vi "Sync.vi"(8 "Input Stream":dbl[](array[numeric]), 9 "error in (no error)":errorcluster, 10 "Frame Instruction":T1, 11 "PN sequence order (9)":i32=9) -> (0 "number 2":u32, 1 "number":u32, 2 "error out":errorcluster)   [LabVIEW 2014]
uses:
  <vilib>/addons/Modulation/Digital/General/MT Generate Bits (Galois, PN Order).vi
  <vilib>/addons/Modulation/Digital/Support/Common/Validators/mod_Generate Bits Validate.vi
  <vilib>/addons/Modulation/Analog/support/mod_Set Error Source.vi
  <vilib>/addons/Modulation/Digital/General/subVIs/mod_Generate Bits PN Sequence.vi
  <vilib>/addons/Modulation/niDMT.lvlib
panel:
  out "Numeric":dbl
  out "output bit stream":i8[](array[numeric])
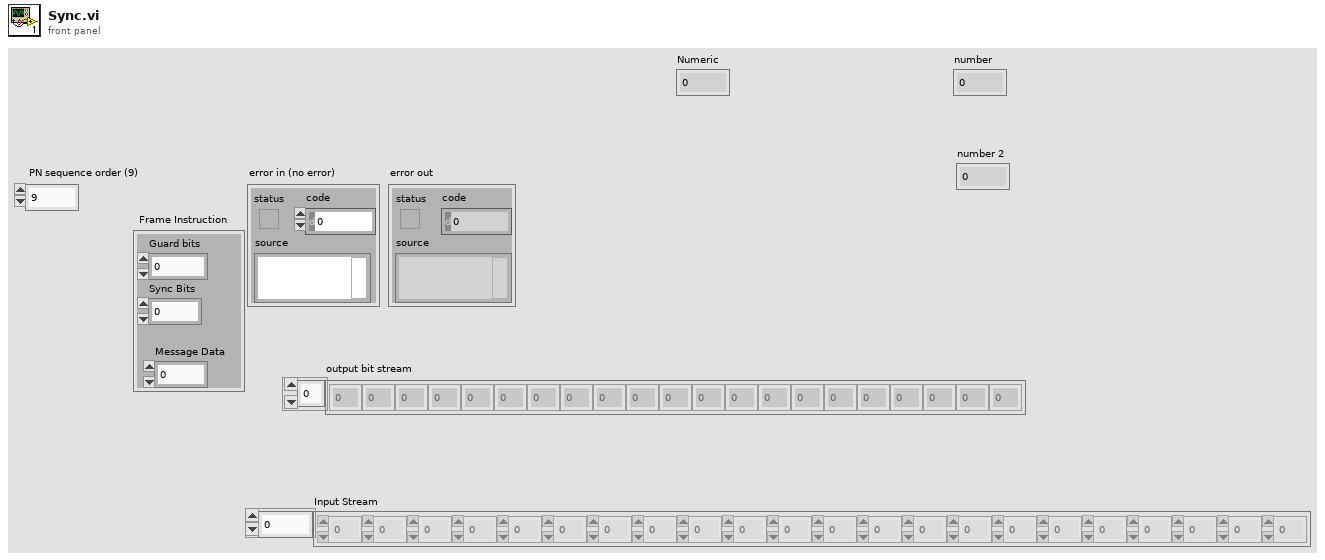
[diagram p1: front panel]
types:
  T1 = cluster{"Guard bits":dbl, "Sync Bits":dbl, "Message Data":dbl}
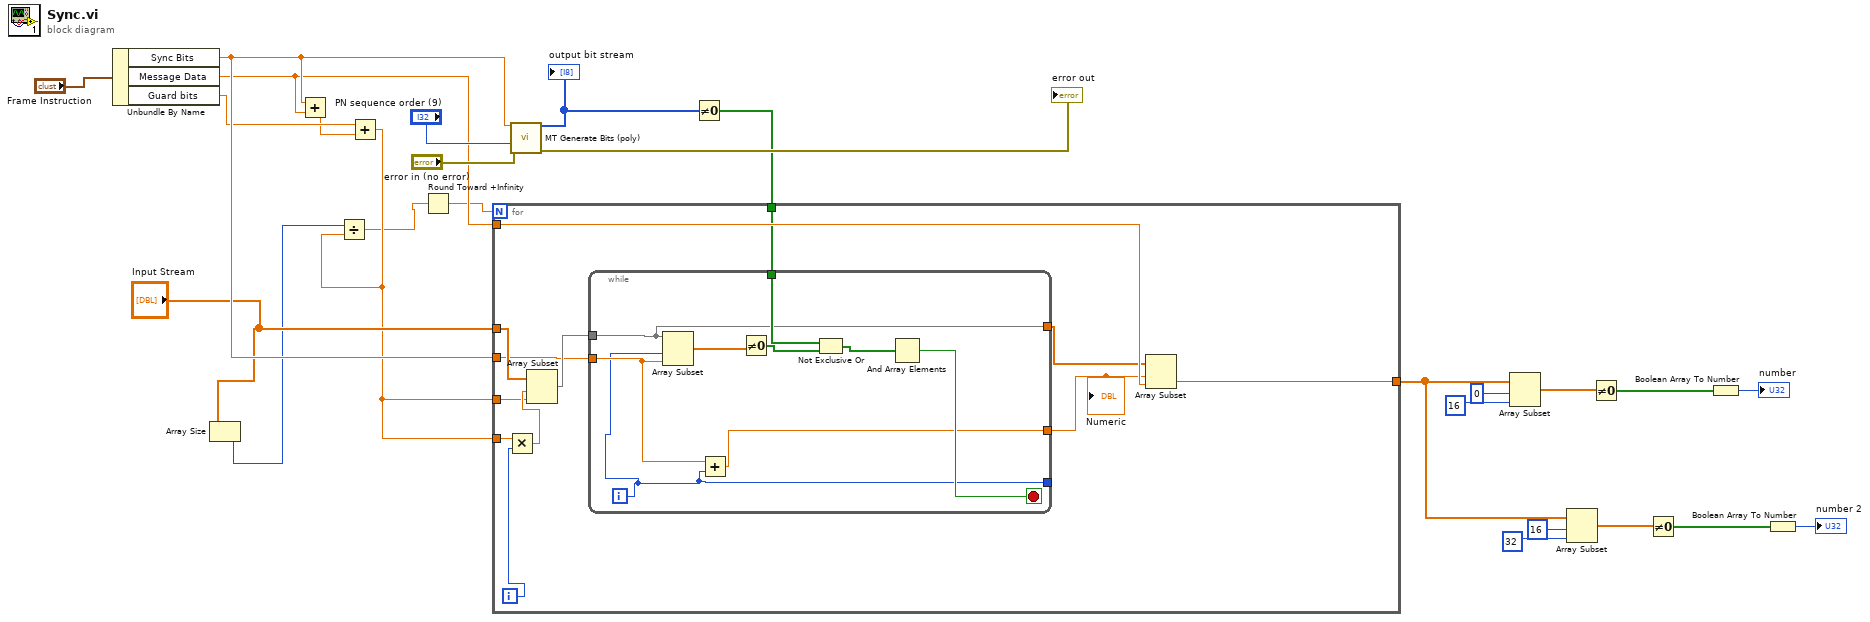
[diagram p0: block diagram]
diagram:
  n1 = Unbundle By Name("Frame Instruction") -> ("Sync Bits"=w22:dbl, "Message Data"=w20:dbl, "Guard bits"=w21:dbl)
  n2 = Array Size(array="Input Stream") -> (size(s)=w18:i32)
  n3 = Add(x=w22, y=w20) -> (x+y=w12:dbl)
  n4 = Add(x=w21, y=w12) -> (x+y=w17:dbl)
  n5 = Divide(x=w18, y=w17) -> (x/y=w16:dbl)
  n6 = Round Toward +Infinity(x=w16) -> (ceil(x): smallest int >= x=w15:dbl)
  n7 = call-poly <vilib>:"MT Generate Bits (poly).vi"("total bits (128)"=w22, "PN sequence order (9)"="PN sequence order (9)", "error in (no error)"="error in (no error)") -> ("output bit stream"=w14:i8[], "error out"=→"error out":errorcluster)  [unwired: 10 in, 1 out]
  "output bit stream" <- w14
  n8 = Not Equal To 0?(x=w14) -> (x != 0?=w13:bool[])
  n9 = for {
    N: w15 -> [_]
    tunnel: "Input Stream" -> [w35]
    tunnel: w22 -> [w30]
    tunnel: w20 -> [w34]
    tunnel: w17 -> [w37]
    tunnel: w17 -> [w33]
    tunnel: w13 -> [w32]
    tunnel: [w27] -> w1
    i -> [w38]
    n10 = Multiply(x=w37, y=w38) -> (x*y=w36:dbl)
    n11 = Array Subset(array=w35, index=w36, length=w33) -> (w31:dbl[])
    n12 = while {
      tunnel: w31 -> [w42]
      tunnel: w30 -> [w41]
      tunnel: w32 -> [w46]
      tunnel: [w42] -> w29
      tunnel: [w40] -> w28
      tunnel: [w39] -> _
      i -> [w39]
      stop <- w43 stop-if-true
      n13 = Array Subset(array=w42, index=w39, length=w41) -> (w47:dbl[])
      n14 = Add(x=w41, y=w39) -> (x+y=w40:dbl)
      n15 = Not Equal To 0?(x=w47) -> (x != 0?=w45:bool[])
      n16 = Not Exclusive Or(1:w45, 2:w46) -> (0:w44:bool[])
      n17 = And Array Elements(Boolean array=w44) -> (logical AND=w43:bool)
    }
    "Numeric" <- w28
    n18 = Array Subset "Array Subset"(array=w29, index=w28, length=w34) -> (w27:dbl[])
  }
  n19 = Array Subset(array=w1, index=0, length=16) -> (w9:dbl[])
  n20 = Array Subset(array=w1, index=16, length=32) -> (w4:dbl[])
  n21 = Not Equal To 0?(x=w9) -> (x != 0?=w8:bool[])
  n22 = Not Equal To 0?(x=w4) -> (x != 0?=w3:bool[])
  n23 = Boolean Array To Number(Boolean array=w8) -> (number=→"number":u32)
  n24 = Boolean Array To Number(Boolean array=w3) -> (number=→"number 2":u32)
